vi "Cancel Error From List.vi"(7 "Codes to Ignore":i32[](array[numeric]), 10 "error in (no error)":errorcluster) -> (2 "error out":errorcluster)   [LabVIEW 2017]
panel:
  # "This VI is used to ignore a group of errors."
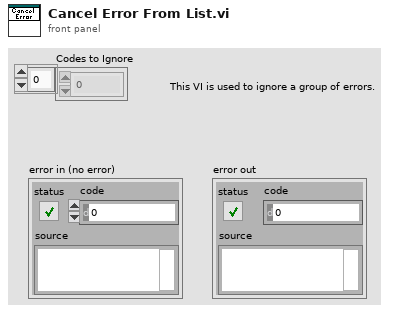
[diagram p1: front panel]
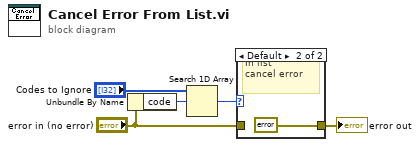
[diagram p0: block diagram]
diagram:
  n1 = Unbundle By Name("error in (no error)") -> ("code"=w2:i32)
  n2 = Search 1D Array(1D array="Codes to Ignore", element=w2) -> (index of element=w3:i32)  [unwired: 1 in]
  n3 = case shown="Default" w3 {
    tunnel: [w6 errorcluster {"status"=FALSE, "code"=0, "source"=""} ("error out")] -> w5
    tunnel: "error in (no error)" -> [w6 _]
    frame -1 {
      # "Not in list \npass thru"
    }
    frame Default {
      # "In list \ncancel error"
    }
  }
  "error out" <- w5
